vi "For索引隧道.vi"() -> ()   [LabVIEW 2014]
panel:
  out "输出数值":dbl
  in  "输入数值":dbl=20.0
  out "循环次数2":i32
  out "数组元素2":i32
  out "循环次数1":i32
  out "数组大小":i32
  out "数组":i32[](array[numeric])
  out "数组元素1":i32
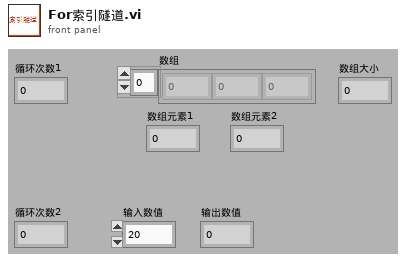
[diagram p1: front panel]
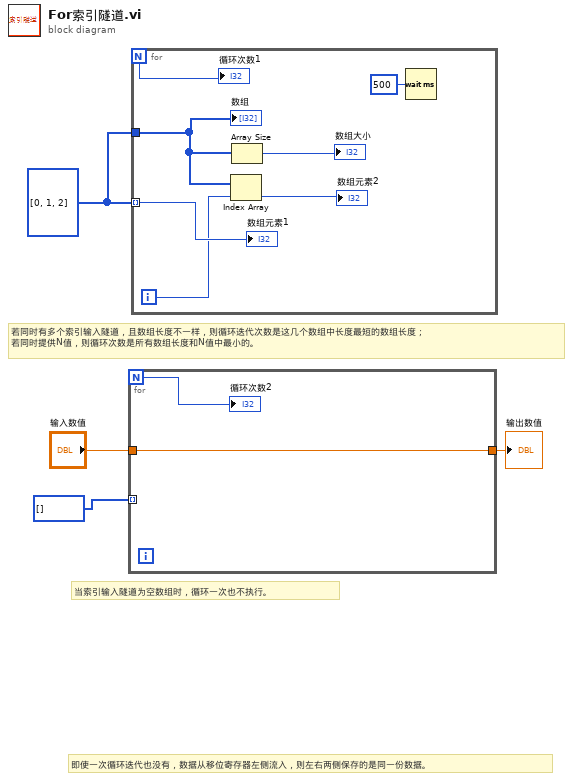
[diagram p0: block diagram]
diagram:
  w4 = i32[] [0, 1, 2]
  # "即使一次循环迭代也没有，数据从移位寄存器左侧流入，则左右两侧保存的是同一份数据。"
  # "当索引输入隧道为空数组时，循环一次也不执行。"
  # "若同时有多个索引输入隧道，且数组长度不一样，则循环迭代次数是这几个数组中长度最短的数组长度；\n若同时提供N值，则循环次数是所有数组长度和N值中最小的。"
  n1 = for {
    N -> [w6]
    tunnel: i32[] [] -> [_] mode=indexing
    tunnel: "输入数值" -> [w5]
    tunnel: [w5] -> w2
    "循环次数2" <- w6
  }
  "输出数值" <- w2
  n2 = for {
    N -> [w11]
    tunnel: w4 -> [w13] mode=indexing
    tunnel: w4 -> [w10]
    i -> [w9]
    n3 = Index Array(array=w10, index=w9) -> (element=→"数组元素2":i32)
    n4 = Array Size(array=w10) -> (size(s)=→"数组大小":i32)
    n5 = Wait (ms)(milliseconds to wait=u32 500 ("等待时间（毫秒）")) -> ()  [unwired: 1 out]
    "数组元素1" <- w13
    "数组" <- w10
    "循环次数1" <- w11
  }
